vi "module-05-sample-5-1-Alt.vi"() -> ()   [LabVIEW 2019]
uses:
  <vilib>/Rock Robotics/WPI/ThirdParty/JAS_Junk/TrajLib/Timer_New.vi
  <vilib>/Rock Robotics/WPI/ThirdParty/JAS_Junk/TrajLib/Timer_Start.vi
  <vilib>/Rock Robotics/WPI/ThirdParty/JAS_Junk/TrajLib/Timer_HasPeriodPassedOnce.vi
  samples-common-library/Ctrl_Training_Library_Protected/CtrlTrainingLibary_Protected.lvlib
  <vilib>/Rock Robotics/WPI/ThirdParty/JAS_Junk/TrajLib/Trajectory_Library.lvlib
panel:
  in  "Tab Control":enum32{"Execution", "Logic"}(tab)
  in  "Driver Gather Cube":bool
  in  "Driver Cancel Button":bool
  out "Request GO":bool
  out "Digital State Chart":cluster{dbl, dbl, dbl, dbl, dbl, dbl}(graph)
  out "Ready":bool
  out "Arm Extend Cmd":bool
  out "Hand Close Cmd":bool
  out "Cur Time":dbl format="%20.3f"
  # "Training Sample 5.1 Alt\nSequential Logic\n    (Enhanced Cancel)"
  # "F1"
  # "F2"
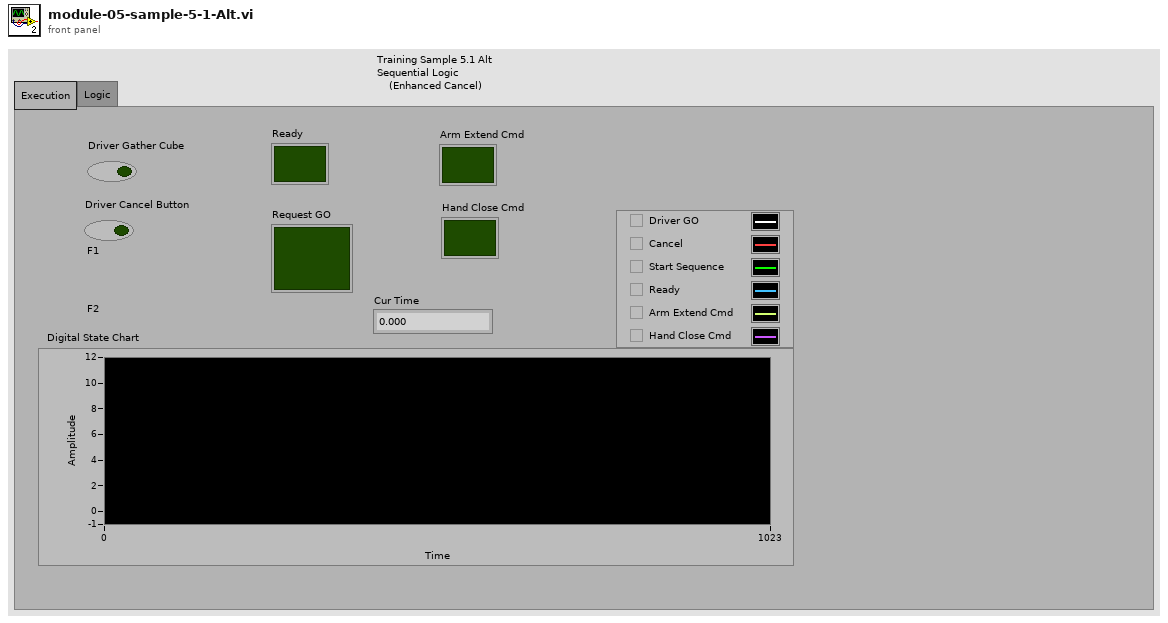
[diagram p1: front panel]
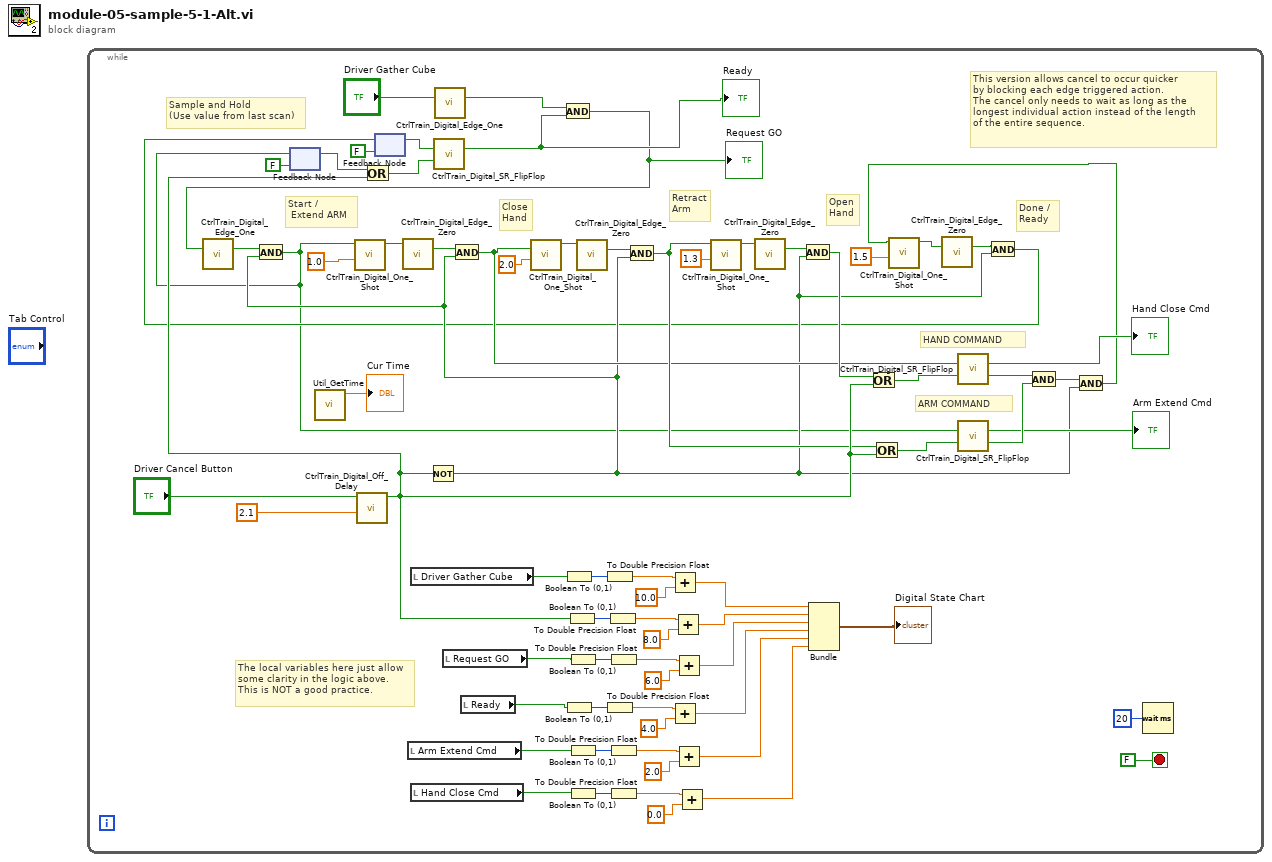
[diagram p0: block diagram]
diagram:
  n1 = while {
    stop <- FALSE stop-if-true
    # "The local variables here just allow\nsome clarity in the logic above.\nThis is NOT a good practice."
    # "Sample and Hold\n(Use value from last scan)"
    # "This version allows cancel to occur quicker\nby blocking each edge triggered action.\nThe cancel only needs to wait as long as the \nlongest individual action instead of the length\nof the entire sequence."
    # "Done / \nReady"
    # "Open\nHand"
    # "Retract\nArm"
    # "Close\nHand"
    # "Start /\n Extend ARM"
    # "HAND COMMAND"
    # "ARM COMMAND"
    n2 = feedback #1(FALSE ("Arm Extend Cmd")) -> (w3:bool)
    n3 = call <vilib>:"Util_GetTime.vi"() -> ("FPGA_Time_Seconds"=→"Cur Time":dbl)  [unwired: 10 in, 1 out]
    n4 = call "CtrlTrain_Digital_Off_Delay.vi"("Delay"=2.1 ("OneShot"), "Input"="Driver Cancel Button") -> ("Output"=w19:bool)  [unwired: 8 in, 1 out]
    n5 = Or(x=w3, y=w19) -> (x .or. y?=w22:bool)
    n6 = feedback #2(FALSE ("Arm Extend Cmd")) -> (w5:bool)
    n7 = local read "Arm Extend Cmd"() -> (w26:bool)
    n8 = local read "Driver Gather Cube"() -> (w30:bool)
    n9 = local read "Hand Close Cmd"() -> (w27:bool)
    n10 = Not(x=w19) -> (.not. x?=w9:bool)
    n11 = call "CtrlTrain_Digital_SR_FlipFlop.vi"("Set"=w5, "Reset"=w22) -> ("Output"=w25:bool)  [unwired: 12 in, 1 out]
    "Ready" <- w25
    n12 = call "CtrlTrain_Digital_Edge_One.vi"("Input"="Driver Gather Cube") -> ("Output"=w20:bool)  [unwired: 14 in]
    n13 = local read "Request GO"() -> (w24:bool)
    n14 = local read "Ready"() -> (w23:bool)
    n15 = And(x=w20, y=w25) -> (x .and. y?=w18:bool)
    "Request GO" <- w18
    n16 = call "CtrlTrain_Digital_Edge_One.vi"("Input"=w18) -> ("Output"=w10:bool)  [unwired: 14 in]
    n17 = And(x=w10, y=w9) -> (x .and. y?=w2:bool)
    n18 = feedback-in #1(w2) -> ()
    n19 = call "CtrlTrain_Digital_One_Shot.vi"("OneShot"=1.0, "Input"=w2) -> ("Output"=w44:bool)  [unwired: 8 in, 1 out]
    n20 = call "CtrlTrain_Digital_Edge_Zero.vi"("Input"=w44) -> ("Output"=w11:bool)  [unwired: 14 in]
    n21 = And(x=w11, y=w9) -> (x .and. y?=w12:bool)
    n22 = call "CtrlTrain_Digital_One_Shot.vi"("OneShot"=2.0, "Input"=w12) -> ("Output"=w43:bool)  [unwired: 8 in, 1 out]
    n23 = Boolean To (0,1)(Boolean=w30) -> (0, 1=w70:i16)
    n24 = Boolean To (0,1)(Boolean=w23) -> (0, 1=w68:i16)
    n25 = Boolean To (0,1)(Boolean=w19) -> (0, 1=w65:i16)
    n26 = Boolean To (0,1)(Boolean=w24) -> (0, 1=w62:i16)
    n27 = Boolean To (0,1)(Boolean=w26) -> (0, 1=w59:i16)
    n28 = Boolean To (0,1)(Boolean=w27) -> (0, 1=w56:i16)
    n29 = call "CtrlTrain_Digital_Edge_Zero.vi"("Input"=w43) -> ("Output"=w14:bool)  [unwired: 14 in]
    n30 = To Double Precision Float(number=w70) -> (double precision float=w47:dbl)
    n31 = To Double Precision Float(number=w68) -> (double precision float=w67:dbl)
    n32 = To Double Precision Float(number=w65) -> (double precision float=w64:dbl)
    n33 = To Double Precision Float(number=w62) -> (double precision float=w61:dbl)
    n34 = To Double Precision Float(number=w59) -> (double precision float=w58:dbl)
    n35 = To Double Precision Float(number=w56) -> (double precision float=w55:dbl)
    n36 = And(x=w14, y=w9) -> (x .and. y?=w13:bool)
    n37 = Add(x=w47, y=10.0) -> (x+y=w46:dbl)
    n38 = Add(x=w67, y=4.0) -> (x+y=w50:dbl)
    n39 = Add(x=w64, y=8.0) -> (x+y=w52:dbl)
    n40 = Add(x=w61, y=6.0) -> (x+y=w51:dbl)
    n41 = Add(x=w58, y=2.0) -> (x+y=w54:dbl)
    n42 = Add(x=w55, y=0.0) -> (x+y=w53:dbl)
    n43 = call "CtrlTrain_Digital_One_Shot.vi"("OneShot"=1.3, "Input"=w13) -> ("Output"=w42:bool)  [unwired: 8 in, 1 out]
    n44 = call "CtrlTrain_Digital_Edge_Zero.vi"("Input"=w42) -> ("Output"=w15:bool)  [unwired: 14 in]
    n45 = And(x=w15, y=w9) -> (x .and. y?=w16:bool)
    n46 = Bundle(w46, w52, w51, w50, w54, w53) -> (→"Digital State Chart":cluster{dbl, dbl, dbl, dbl, dbl, dbl})  [unwired: 1 in]
    n47 = Or(x=w16, y=w19) -> (x .or. y?=w33:bool)
    n48 = Or(x=w13, y=w19) -> (x .or. y?=w32:bool)
    n49 = call "CtrlTrain_Digital_SR_FlipFlop.vi"("Set"=w12, "Reset"=w33) -> ("Output"=→"Hand Close Cmd":bool, "Inverse Output"=w36:bool)  [unwired: 12 in]
    n50 = call "CtrlTrain_Digital_SR_FlipFlop.vi"("Set"=w2, "Reset"=w32) -> ("Output"=→"Arm Extend Cmd":bool, "Inverse Output"=w37:bool)  [unwired: 12 in]
    n51 = And(x=w36, y=w37) -> (x .and. y?=w31:bool)
    n52 = And(x=w31, y=w9) -> (x .and. y?=w8:bool)
    n53 = call "CtrlTrain_Digital_One_Shot.vi"("OneShot"=1.5, "Input"=w8) -> ("Output"=w41:bool)  [unwired: 8 in, 1 out]
    n54 = call "CtrlTrain_Digital_Edge_Zero.vi"("Input"=w41) -> ("Output"=w17:bool)  [unwired: 14 in]
    n55 = And(x=w17, y=w9) -> (x .and. y?=w4:bool)
    n56 = feedback-in #2(w4) -> ()
    n57 = Wait (ms)(milliseconds to wait=u32 20) -> ()  [unwired: 1 out]
  }
